vi "Set CAN Adapters.vi"(10 "CAN Adapters":refnum<class "ICAN.lvclass">[](array[class]), 11 "Interactor in":refnum<class "Interactor.lvclass">) -> (3 "Interactor out":refnum<class "Interactor.lvclass">)   [LabVIEW 2024, in "Interactor.lvlib" / "Interactor.lvclass"]
uses:
  Interactor.lvclass
  Interactor.lvclass/Interactor.ctl
  HAL/HAL/Protocols/ICAN/ICAN.lvclass
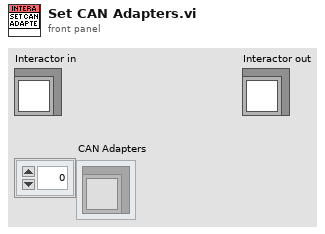
[diagram p1: front panel]
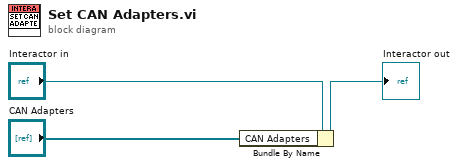
[diagram p0: block diagram]
diagram:
  n1 = Bundle By Name(cluster="Interactor in", "CAN Adapters"="CAN Adapters") -> (→"Interactor out":refnum<class "Interactor.lvclass">)
